vi "Get Text With Markdown.vi"(8 "error in":errorcluster, 11 "Free Label Ref":refnum<vi>) -> (0 "error out":errorcluster, 1 "Processing Time (ms)":u32, 2 "Text (no markdown)":string, 3 "Text (with markdown)":string)   [LabVIEW 2016]
panel:
  out "Class Name":string
  out "Property Node Execution Time (ms)":u32[](array[numeric])
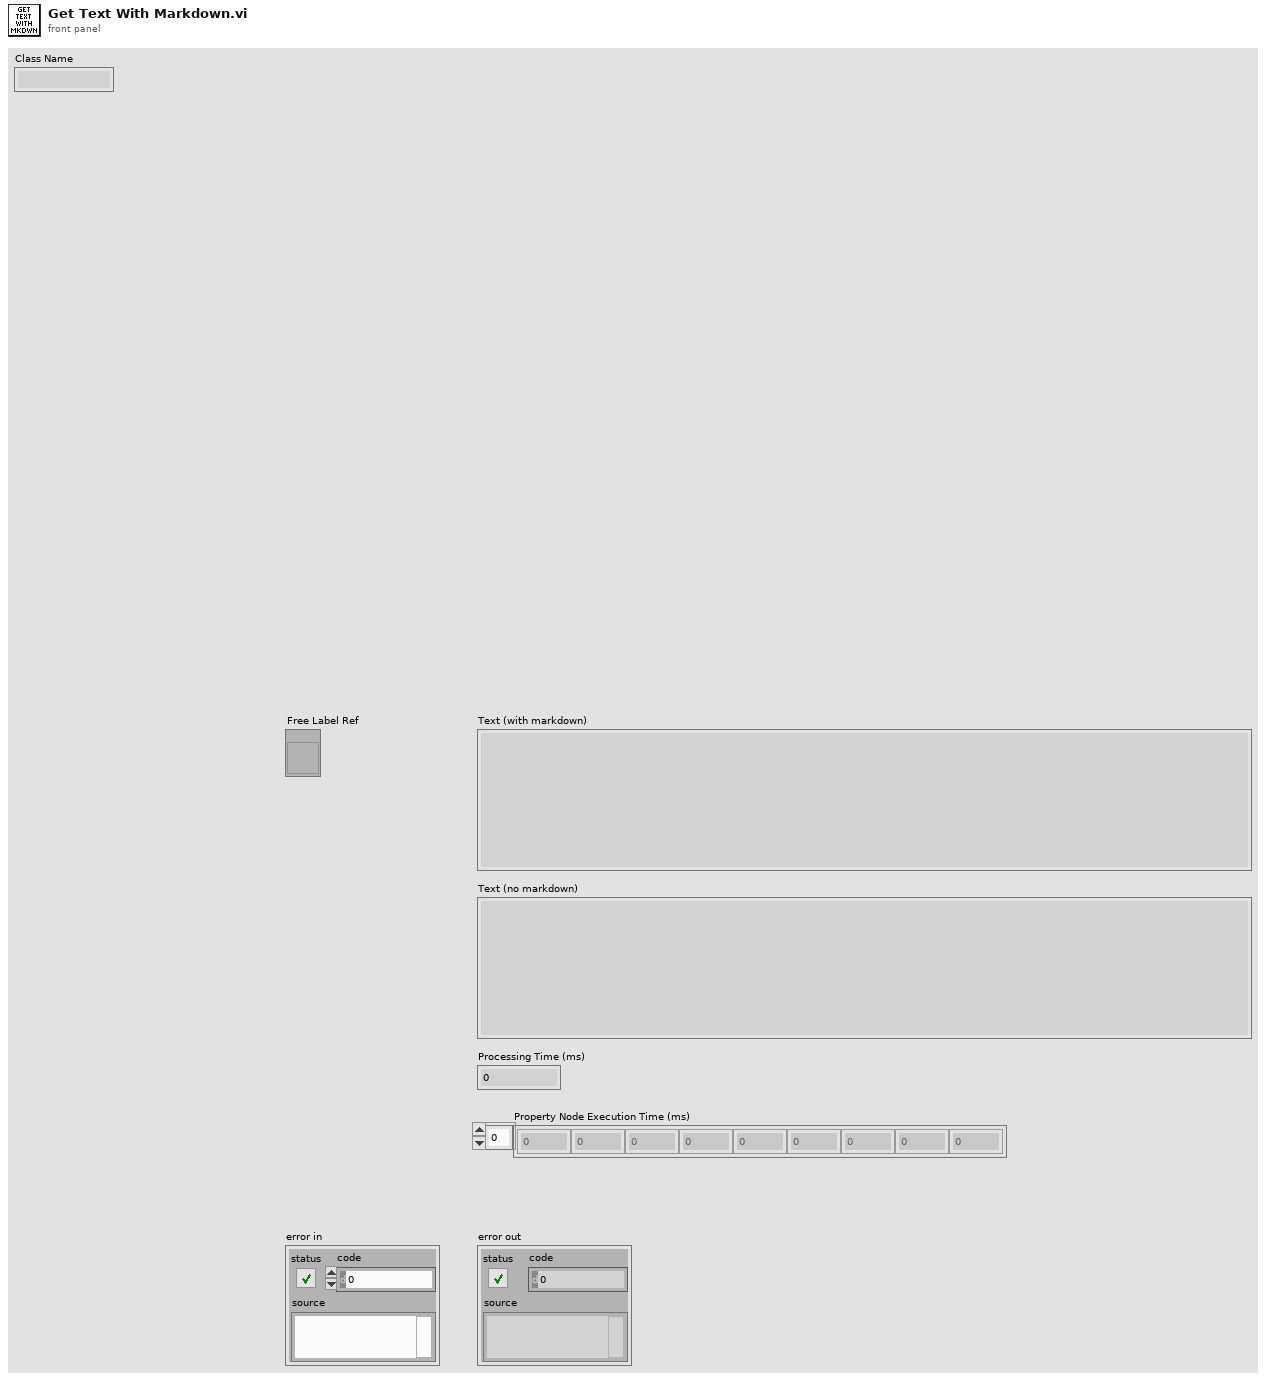
[diagram p1: front panel]
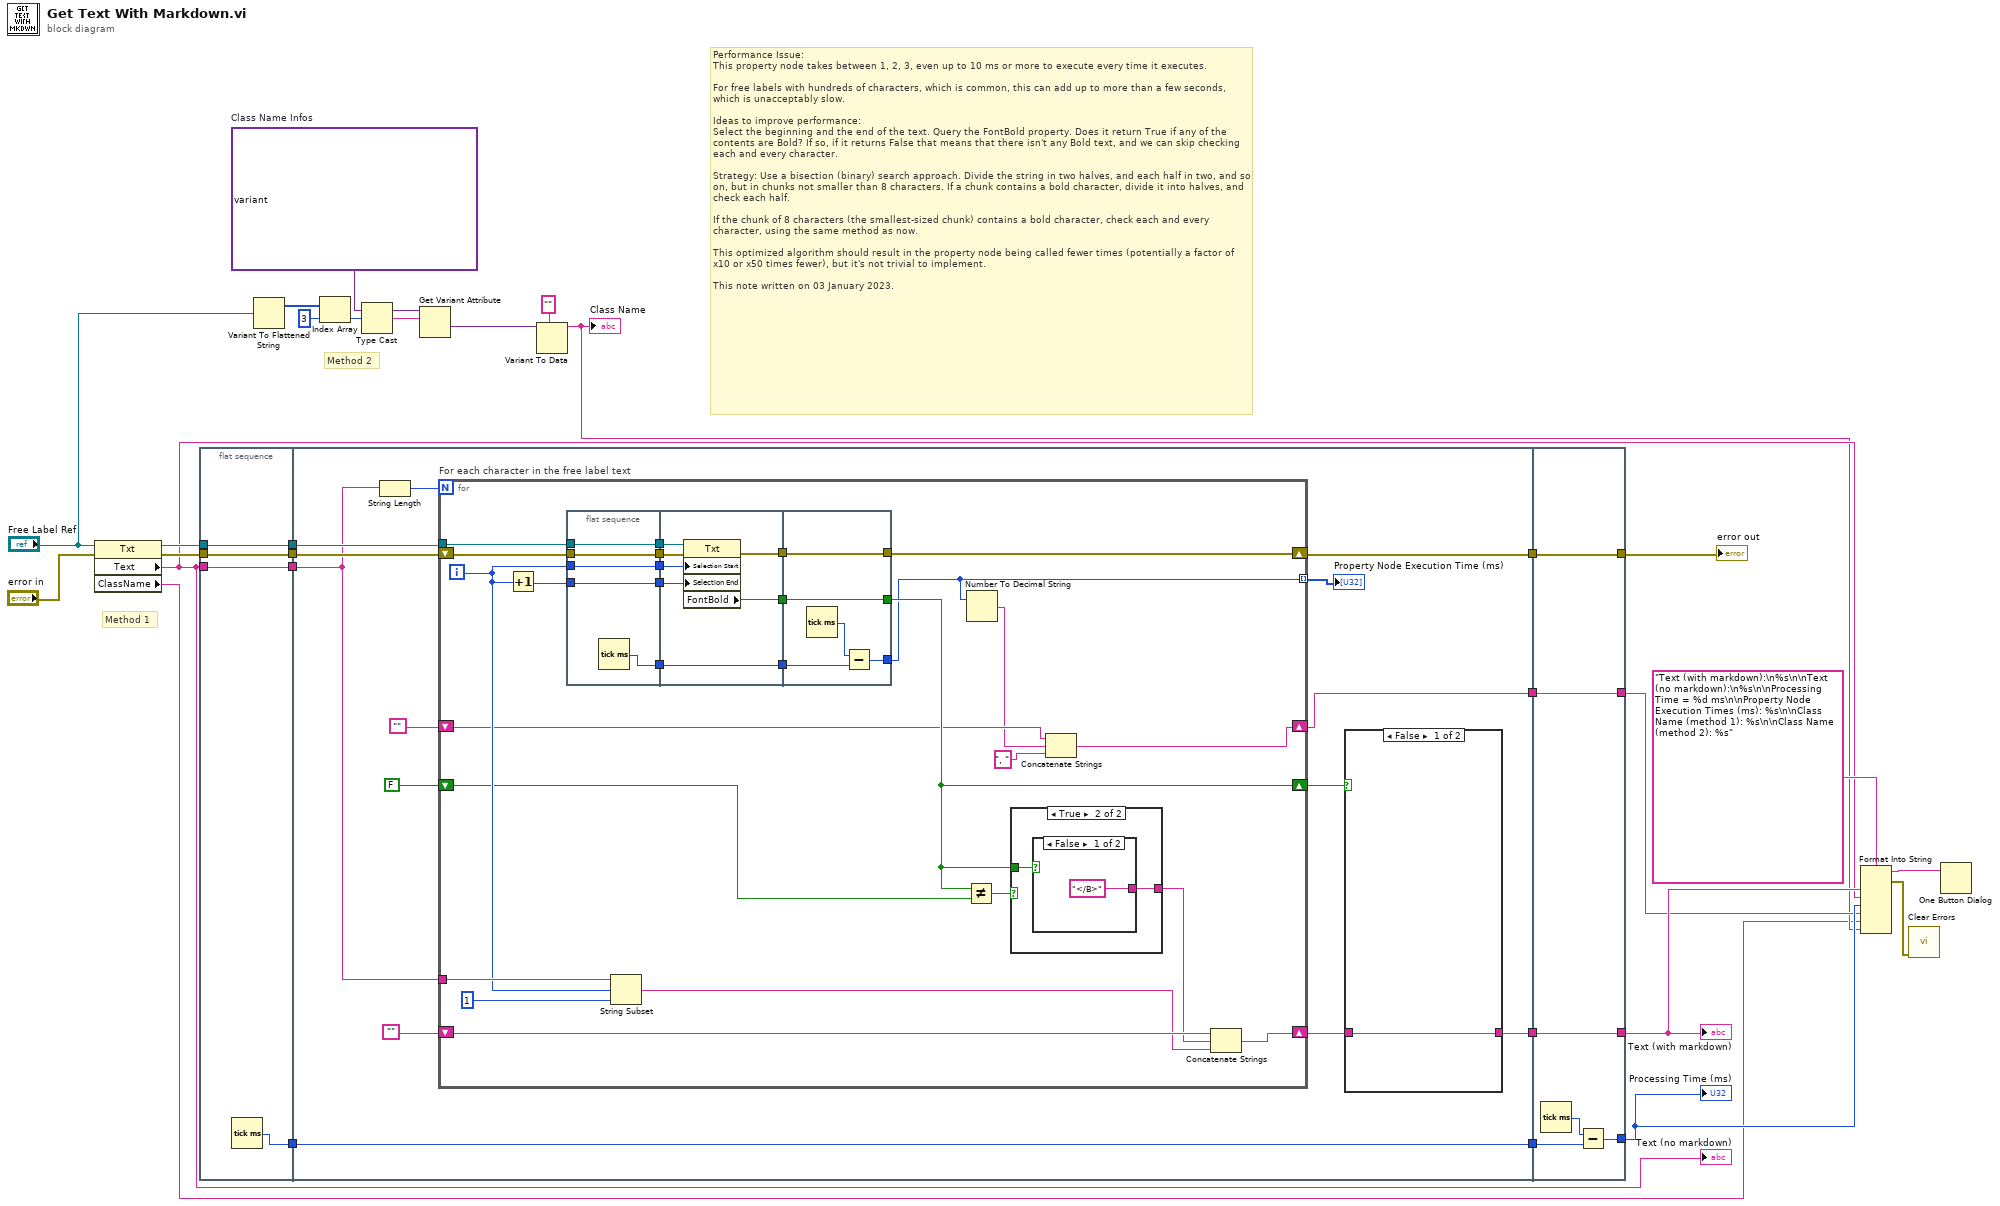
[diagram p0: block diagram]
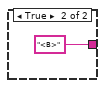
[diagram p3: hidden frame]
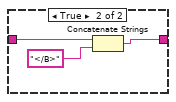
[diagram p4: hidden frame]
diagram:
  w10 = variant("\u0000\u0004"=variant(string "Decoration"), "\u0000\u0005"=variant(string "Text"), "\u0000\u0006"=variant(string "Control"), "\u0000\u0007"=variant(string "ColorBox"), "\u0000\b"=variant(string "Boolean"), "\u0000\t"=variant(string "RefNum"), "\u0000\n"=variant(string "LVVariant"), "\u0000\u000b"=variant(string "Path"), "\u0000\f"=variant(string "ListBox"), "\u0000\r"=variant(string "Table"), "\u0000\u000e"=variant(string "Array"), "\u0000\u000f"=variant(string "Picture"), "\u0000\u0010"=variant(string "ActiveXContainer"), "\u0000\u0011"=variant(string "Numeric"), "\u0000\u0012"=variant(string "Digital"), "\u0000\u0013"=variant(string "NamedNumeric"), "\u0000\u0014"=variant(string "ColorRamp"), "\u0000\u0015"=variant(string "Slide"), "\u0000\u0016"=variant(string "GraphChart"), "\u0000\u0017"=variant(string "WaveformChart"), "\u0000\u0018"=variant(string "WaveformGraph"), "\u0000\u0019"=variant(string "IntensityChart"), "\u0000\u001a"=variant(string "IntensityGraph"), "\u0000\u001b"=variant(string "String"), "\u0000\u001c"=variant(string "IOName"), "\u0000\u001d"=variant(string "ComboBox"), "\u0000\u001e"=variant(string "Cluster"), "\u0000\u001f"=variant(string "Panel"), "\u0000 "=variant(string "Knob"), "\u0000!"=variant(string "NumericWithScale"), "\u0000\""=variant(string "Ring"), "\u0000#"=variant(string "Enum"), "\u0000$"=variant(string "GObject"), "\u0000'"=variant(string "NumericText"), "\u0000("=variant(string "Scale"), "\u0000)"=variant(string "ColorScale"), "\u0000*"=variant(string "GraphScale"), "\u0000+"=variant(string "ColorGraphScale"), "\u0000,"=variant(string "TypedRefNum"), "\u0000."=variant(string "MulticolumnListbox"), "\u0000/"=variant(string "WaveformData"), "\u00000"=variant(string "DSCTag"), "\u00001"=variant(string "DAQChannelName"), "\u00002"=variant(string "VISAResourceName"), "\u00003"=variant(string "IVILogicalName"), "\u00004"=variant(string "SlideScale"), "\u00005"=variant(string "PageSelector"), "\u00007"=variant(string "TabControl"), "\u00009"=variant(string "DAQmxName"), "\u0000:"=variant(string "VIRefNum"), "\u0000;"=variant(string "LVObjectRefNum"), "\u0000<"=variant(string "AbsTime"), "\u0000="=variant(string "DigitalTable"), "\u0000A"=variant(string "SubPanel"), "\u0000B"=variant(string "TreeControl"), "\u0000C"=variant(string "GenClassTagRef"), "\u0000D"=variant(string "GenClassRef"), "\u0000E"=variant(string "RotaryColorScale"), "\u0000F"=variant(string "PlugInControl"), "\u0000G"=variant(string "PlugInDDODummyContainer"), "\u0000H"=variant(string "RadioButtonsControl"), "\u0000K"=variant(string "Pane"), "\u0000L"=variant(string "Splitter"), "\u0000N"=variant(string "Pixmap"), "\u0000S"=variant(string "XYGraph"), "\u0000Z"=variant(string "Scrollbar"), "\u0000\\"=variant(string "MixedSignalGraph"), "\u0000d"=variant(string "SceneGraphDisplay"), "\u0000f"=variant(string "LabVIEWClassControl"), "\u0000y"=variant(string "DigitalGraph"), "\u0000"=variant(string "MixedCheckbox"), "\u0000‚"=variant(string "MultiSegmentPipe"), "\u0000„"=variant(string "StubDDO"), "\u0000‡"=variant(string "DataValRefNum"), "\u0000ˆ"=variant(string "Set"), "\u0000‰"=variant(string "Map"), "@\u0000"=variant(string "Diagram"), "@\u0001"=variant(string "Terminal"), "@\u0002"=variant(string "Constant"), "@\u0003"=variant(string "PathConstant"), "@\u0004"=variant(string "ArrayConstant"), "@\u0005"=variant(string "NumericConstant"), "@\u0006"=variant(string "DigitalNumericConstant"), "@\u0007"=variant(string "NamedNumericConstant"), "@\b"=variant(string "StringConstant"), "@\t"=variant(string "ClusterConstant"), "@\n"=variant(string "FixedConstant"), "@\u000b"=variant(string "ControlTerminal"), "@\f"=variant(string "FormulaParameter"), "@\r"=variant(string "Global"), "@\u000e"=variant(string "Local"), "@\u000f"=variant(string "RightShiftRegister"), "@\u0010"=variant(string "Function"), "@\u0011"=variant(string "SubVI"), "@\u0012"=variant(string "CallByRef"), "@\u0013"=variant(string "UnitCast"), "@\u0014"=variant(string "Structure"), "@\u0015"=variant(string "Loop"), "@\u0016"=variant(string "MultiFrameStructure"), "@\u0017"=variant(string "Sequence"), "@\u0018"=variant(string "CaseStructure"), "@\u0019"=variant(string "Formula"), "@\u001a"=variant(string "GrowableFunction"), "@\u001b"=variant(string "BuildClusterArray"), "@\u001c"=variant(string "CompoundArithmetic"), "@\u001d"=variant(string "IndexArray"), "@\u001e"=variant(string "BuildArray"), "@\u001f"=variant(string "NamedBundler"), "@ "=variant(string "CIN"), "@!"=variant(string "CallLibrary"), "@\""=variant(string "ObjectFunction"), "@#"=variant(string "Property"), "@$"=variant(string "Invoke"), "@%"=variant(string "Node"), "@&"=variant(string "BooleanConstant"), "@'"=variant(string "TopLevelDiagram"), "@("=variant(string "RingConstant"), "@)"=variant(string "EnumConstant"), "@*"=variant(string "Tunnel"), "@+"=variant(string "LoopTunnel"), "@,"=variant(string "SequenceLocal"), "@-"=variant(string "Comparison"), "@."=variant(string "ReadWriteFile"), "@/"=variant(string "TypeCast"), "@0"=variant(string "FlattenUnflattenString"), "@1"=variant(string "GPIBReadWrite"), "@2"=variant(string "ForLoop"), "@3"=variant(string "WhileLoop"), "@4"=variant(string "ScriptNode"), "@5"=variant(string "ArrayToCluster"), "@6"=variant(string "FormatScanString"), "@7"=variant(string "Wire"), "@9"=variant(string "InnerTerminal"), "@:"=variant(string "LeftShiftRegister"), "@;"=variant(string "PolymorphicSubVI"), "@<"=variant(string "PropertyItem"), "@="=variant(string "IONameConstant"), "@>"=variant(string "DSCTagConstant"), "@?"=variant(string "DAQChannelNameConstant"), "@@"=variant(string "VISAResourceNameConstant"), "@A"=variant(string "IVILogicalNameConstant"), "@B"=variant(string "ColorBoxConstant"), "@C"=variant(string "ControlReferenceConstant"), "@D"=variant(string "ClassSpecifierConstant"), "@E"=variant(string "ConfNode"), "@H"=variant(string "OuterTerminal"), "@I"=variant(string "DAQmxNameConstant"), "@J"=variant(string "EventStructure"), "@K"=variant(string "FlatSequence"), "@L"=variant(string "GenClassTagRefConstant"), "@M"=variant(string "AbsTimeConstant"), "@N"=variant(string "ExternalNode"), "@P"=variant(string "ScriptNodeParameter"), "@Q"=variant(string "StaticVIReference"), "@R"=variant(string "ComboBoxConstant"), "@S"=variant(string "TimedLoop"), "@U"=variant(string "GenClassTagFlatRef"), "@V"=variant(string "GenClassTagFlatRefConstant"), "@X"=variant(string "SimDiagram"), "@Y"=variant(string "CompanionDiagram"), "@Z"=variant(string "SimulationNode"), "@["=variant(string "SimulationDCO"), "@\\"=variant(string "Bundler"), "@]"=variant(string "Unbundler"), "@^"=variant(string "NamedUnbundler"), "@`"=variant(string "FlatSequenceInnerTunnel"), "@a"=variant(string "FlatSequenceOuterTunnel"), "@b"=variant(string "RefNumConstant"), "@c"=variant(string "FlattenString"), "@d"=variant(string "PolymorphicVISelector"), "@e"=variant(string "XNode"), "@f"=variant(string "SelectorTunnel"), "@g"=variant(string "DisableStructure"), "@h"=variant(string "SDFDiagram"), "@i"=variant(string "SDF Companion Diagram"), "@j"=variant(string "SynchronousDataFlowNode"), "@k"=variant(string "SynchronousDataFlowDCO"), "@l"=variant(string "FileDialog"), "@m"=variant(string "TimedStructDCO"), "@o"=variant(string "TimeFlatSequence"), "@p"=variant(string "TimedSequence"), "@q"=variant(string "XDataNode"), "@s"=variant(string "MathScriptNode"), "@t"=variant(string "MathScriptNodeParameter"), "@u"=variant(string "LabVIEWClassConstant"), "@v"=variant(string "MathDiagram"), "@w"=variant(string "AbstractDiagram"), "@x"=variant(string "InlineCNode"), "@y"=variant(string "Constructor"), "@z"=variant(string "RegionNode"), "@{"=variant(string "JunctionNode"), "@|"=variant(string "StateNode"), "@}"=variant(string "ForkNode"), "@~"=variant(string "JoinNode"), "@"=variant(string "ScDiagram"), "@€"=variant(string "SharedVariableNode"), "@‚"=variant(string "ParameterTerminal"), "@ƒ"=variant(string "OverridableParameterTerminal"), "@„"=variant(string "InPlaceElementStructure"), "@…"=variant(string "InPlaceBorderNode"), "@†"=variant(string "InPlaceArrayNode"), "@‡"=variant(string "InPlaceClusterNode"), "@ˆ"=variant(string "InPlaceVariantNode"), "@‰"=variant(string "InPlaceElementNode"), "@Š"=variant(string "FeedbackNode"), "@‹"=variant(string "MathScriptCallByRef"), "@Œ"=variant(string "InPlaceDataValRefNode"), "@"=variant(string "ConditionalTunnel"), "@Ž"=variant(string "AbstractDynamicDispatch"), "@"=variant(string "DynamicDispatchSubVI"), "@"=variant(string "CallParentNode"), "@‘"=variant(string "GenClassRefConst"), "@’"=variant(string "InPlaceArraySplitNode"), "@“"=variant(string "SharedVariableDynamicOpen"), "@”"=variant(string "SharedVariableDynamicRead"), "@•"=variant(string "SharedVariableDynamicWrite"), "@–"=variant(string "GenericSubVI"), "@—"=variant(string "InRangeAndCoerce"), "@˜"=variant(string "RegionTunnel"), "@™"=variant(string "StatechartStructureNode"), "@š"=variant(string "TypedRefNumConstant"), "@›"=variant(string "DataValRefNumConstant"), "@œ"=variant(string "TextBaseNode"), "@"=variant(string "ExpressionNode"), "@ž"=variant(string "RegisterForEvents"), "@Ÿ"=variant(string "TargetStructureNode"), "@ "=variant(string "InPlaceVariantAttributeNode"), "@¡"=variant(string "ClosureStructureNode"), "@¢"=variant(string "RaceStructureNode"), "@¤"=variant(string "InPlaceMapNode"), "@¥"=variant(string "BuildSetNode"), "@¦"=variant(string "BuildMapNode"), "@§"=variant(string "AssertStructuralTypeMismatchNode"), "@¨"=variant(string "SetConstant"), "@©"=variant(string "MapConstant"))  # Class Name Infos
  # "Method 2"
  # "Method 1"
  # "Performance Issue:\nThis property node takes between 1, 2, 3, even up to 10 ms or more to execute every time it executes.\n\nFor free labels with hundreds of characters, which is common, this can add up to more than a few seconds, which is unacceptably slow.\n\nIdeas to improve performance:\nSelect the beginning and the end of the text. Query the FontBold property. Does it return True if any of the contents are Bold? If so, if it returns False that means that there isn't any Bold text, and we can skip checking each and every character.\n\nStrategy: Use a bisection (binary) search approach. Divide the string in two halves, and each half in two, and so on, but in chunks not smaller than 8 characters. If a chunk contains a bold character, divide it into halves, and check each half.\n\nIf the chunk of 8 characters (the smallest-sized chunk) contains a bold character, check each and every character, using the same method as now.\n\nThis optimized algorithm should result in the property node being called fewer times (potentially a factor of x10 or x50 times fewer), but it's not trivial to implement.\n\nThis note written on 03 January 2023."
  n1 = property class="Txt"(reference="Free Label Ref", error in="error in") -> (reference out=w29:refnum<vi>, error out=w28:errorcluster, "Text"=w21:string, "ClassName"=w1:string)
  "Text (no markdown)" <- w21
  n2 = flat-sequence {
    tunnel: w21 -> [w31]
    tunnel: w28 -> [w32]
    tunnel: w29 -> [w33]
    tunnel: [w33] -> w18
    tunnel: [w32] -> w17
    tunnel: [w31] -> w16
    tunnel: [w30] -> w14
    tunnel: [w42] -> w20
    tunnel: [w39] -> w19
    tunnel: w18 -> [w47]
    tunnel: w17 -> [w43]
    tunnel: w16 -> [w38]
    tunnel: [w37] -> w15
    tunnel: w14 -> [w37]
    tunnel: [w34] -> w11
    tunnel: [w104] -> w22
    tunnel: [w105] -> w26
    tunnel: w20 -> [w105]
    tunnel: w19 -> [w104]
    tunnel: w15 -> [w102]
    tunnel: [w101] -> w13
    tunnel: [w100] -> w12
    tunnel: w11 -> [w100]
    frame #0 {
      n3 = Tick Count (ms)() -> (millisecond timer value=w30:u32)
    }
    frame #1 {
      n4 = String Length(string=w38) -> (length=w46:i32)
      n5 = for "For each character in the free label text" {
        N: w46 -> [_]
        tunnel: w47 -> [w74]
        tunnel: w38 -> [w71]
        shift-right: [w63] -> w40
        shift-left: "" -> [w66]
        shift-right: [w67] -> w41
        shift-left: FALSE ("Font:Bold") -> [w69]
        shift-right: [w61] -> w42
        shift-left: w43 -> [w62]
        tunnel: [w52] -> w36 mode=indexing
        shift-right: [w48] -> w34
        shift-left: "" -> [w51]
        i -> [w70]
        n6 = Increment(x=w70) -> (x+1=w73:i32)
        n7 = flat-sequence {
          tunnel: w62 -> [w76]
          tunnel: w70 -> [w77]
          tunnel: w73 -> [w78]
          tunnel: w74 -> [w79]
          tunnel: [w79] -> w60
          tunnel: [w78] -> w59
          tunnel: [w77] -> w58
          tunnel: [w76] -> w57
          tunnel: [w75] -> w54
          tunnel: w60 -> [w86]
          tunnel: w59 -> [w85]
          tunnel: w58 -> [w84]
          tunnel: w57 -> [w82]
          tunnel: [w83] -> w56
          tunnel: [w81] -> w55
          tunnel: w54 -> [w80]
          tunnel: [w80] -> w53
          tunnel: [w90] -> w61
          tunnel: [w91] -> w67
          tunnel: w56 -> [w91]
          tunnel: w55 -> [w90]
          tunnel: w53 -> [w88]
          tunnel: [w87] -> w52
          frame #0 {
            n8 = Tick Count (ms)() -> (millisecond timer value=w75:u32)
          }
          frame #1 {
            n9 = property class="Txt"(reference=w86, error in=w82, "Selection Start"=w84, "Selection End"=w85) -> (error out=w81:errorcluster, "FontBold"=w83:bool)  [unwired: 1 out]
          }
          frame #2 {
            n10 = Tick Count (ms)() -> (millisecond timer value=w89:u32)
            n11 = Subtract(x=w89, y=w88) -> (x-y=w87:u32)
          }
        }
        n12 = String Subset(string=w71, offset (0)=w70, length (rest)=1 ("length (rest)")) -> (substring=w64:string)
        n13 = Not Equal?(x=w67, y=w69) -> (x != y?=w68:bool)
        n14 = Number To Decimal String(number=w52) -> (decimal integer string=w50:string)  [unwired: 1 in]
        n15 = case shown="True" w68 {
          tunnel: w67 -> [_ w93]
          tunnel: [_ w92] -> w65
          frame False {
          }
          frame True {
            n16 = case shown="False" w93 {
              tunnel: ["</B>" "<B>"] -> w92
              frame False {
              }
              frame True {
              }
            }
          }
        }
        n17 = Concatenate Strings(w51, w50, ", ") -> (w48:string)
        n18 = Concatenate Strings(w66, w65, w64) -> (w63:string)
      }
      "Property Node Execution Time (ms)" <- w36
      n19 = case shown="False" w41 {
        tunnel: w40 -> [w96 w99]
        tunnel: [w96 w97] -> w39
        frame False {
        }
        frame True {
          n20 = Concatenate Strings(w99, "</B>") -> (w97:string)
        }
      }
    }
    frame #2 {
      n21 = Tick Count (ms)() -> (millisecond timer value=w103:u32)
      n22 = Subtract(x=w103, y=w102) -> (x-y=w101:u32)
    }
  }
  n23 = Variant To Flattened String(Variant="Free Label Ref") -> (1:w9:i16[])  [unwired: 1 out]
  n24 = Index Array(array=w9, index=3) -> (element=w7:i16)
  n25 = Type Cast(x=w7) -> (*(type *) &x=w6:string)  [unwired: 1 in]
  n26 = Get Variant Attribute(Variant=w10, name=w6) -> (value=w5:variant)  [unwired: 2 in, 3 out]
  n27 = Variant To Data(type="", Variant=w5) -> (data=w2:string)  [unwired: 1 in, 1 out]
  "Class Name" <- w2
  n28 = Format Into String(format string="Text (with markdown):\n%s\n\nText (no markdown):\n%s\n\nProcessing Time = %d ms\n\nProperty Node Execution Times (ms): %s\n\nClass Name (method 1): %s\n\nClass Name (method 2): %s", w22, w21, w13, w12, w1, w2) -> (resulting string=w24:string, error out=w23:errorcluster)  [unwired: 2 in]
  n29 = call <vilib>:"Clear Errors.vi"("error in (no error)"=w23) -> ()  [unwired: 5 in, 2 out]
  n30 = One Button Dialog(message=w24) -> ()  [unwired: 1 in, 1 out]
  "Text (with markdown)" <- w22
  "error out" <- w26
  "Processing Time (ms)" <- w13
